vi "GDSProject_GetChidrenItemFromName.vi"(0 "ProjectItemToSearchFrom":refnum<vi>, 1 "ItemNameToSearchForInProjectTree":string, 2 "ItemToSearchForInProjectTreeBasedOnPath(used if wired)":path, 5 "error in (no error)":errorcluster) -> (14 "ProjectItemToSearchFromOut":refnum<vi>, 15 "ItemFound":bool, 16 "ProjectItemFound":refnum<vi>, 19 "error out":errorcluster)   [LabVIEW 2020]
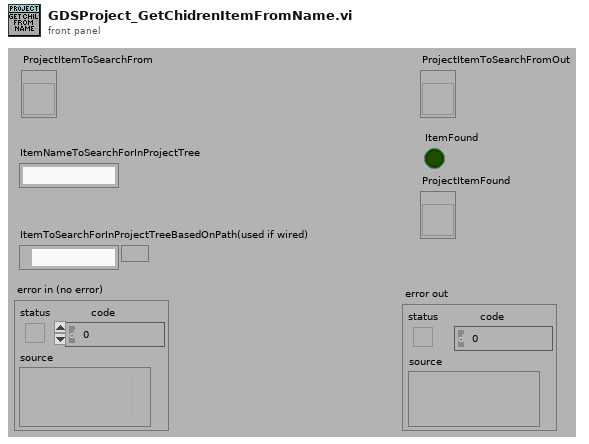
[diagram p1: front panel]
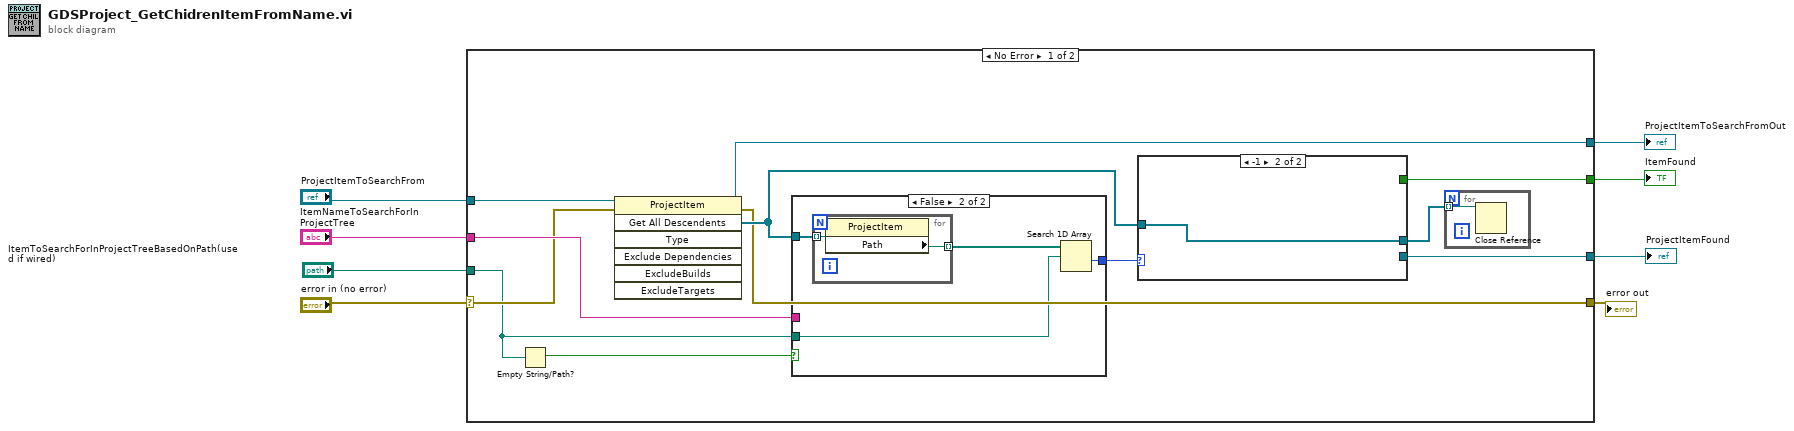
[diagram p0: block diagram]
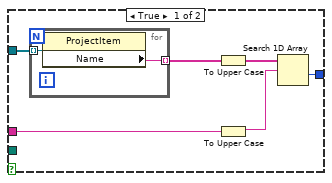
[diagram p2: hidden frame]
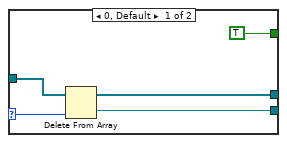
[diagram p3: hidden frame]
diagram:
  n1 = case shown="No Error" "error in (no error)" {
    selector: "error in (no error)" -> [w15 w43]
    tunnel: [w12 w43] -> w7
    tunnel: "ProjectItemToSearchFrom" -> [w20 w42]
    tunnel: "ItemNameToSearchForInProjectTree" -> [w19 _]
    tunnel: [w17 _] -> w4
    tunnel: [w16 w42] -> w3
    tunnel: [w13 _] -> w2
    tunnel: "ItemToSearchForInProjectTreeBasedOnPath(used if wired)" -> [w9 _]
    frame No Error {
      n2 = Empty String/Path?(string/path=w9) -> (empty?=w10:bool)
      n3 = invoke class="ProjectItem" method="Get All Descendents"(reference=w20, error in=w15) -> (reference out=w16:refnum<vi>, error out=w12:errorcluster, "All Descendents"=w14:refnum<vi>[])  [unwired: 5 in, 4 out]
      n4 = case shown="False" w10 {
        tunnel: w19 -> [w25 _]
        tunnel: [w22 w32] -> w18
        tunnel: w14 -> [w21 w31]
        tunnel: w9 -> [_ w29]
        frame True {
          n5 = for {
            tunnel: w21 -> [w28] mode=indexing
            tunnel: [w27] -> w26 mode=indexing
            n6 = property class="ProjectItem"(reference=w28) -> ("Name"=w27:string)  [unwired: 1 in, 2 out]
          }
          n7 = To Upper Case(1:w26) -> (0:w24:string[])
          n8 = To Upper Case(1:w25) -> (0:w23:string)
          n9 = Search 1D Array(1D array=w24, element=w23) -> (index of element=w22:i32)  [unwired: 1 in]
        }
        frame False {
          n10 = for {
            tunnel: w31 -> [w34] mode=indexing
            tunnel: [w33] -> w30 mode=indexing
            n11 = property class="ProjectItem"(reference=w34) -> ("Path"=w33:path)  [unwired: 1 in, 2 out]
          }
          n12 = Search 1D Array(1D array=w30, element=w29) -> (index of element=w32:i32)  [unwired: 1 in]
        }
      }
      n13 = case shown="-1" w18 {
        selector: w18 -> [w38 _]
        tunnel: [TRUE _] -> w17
        tunnel: w14 -> [w39 w41]
        tunnel: [w37 w41] -> w11
        tunnel: [w36 _] -> w13
        frame 0, Default {
          n14 = Delete From Array(array=w39, index=w38) -> (deleted portion=w36:refnum<vi>, array with subset deleted=w37:refnum<vi>[])  [unwired: 1 in]
        }
        frame -1 {
        }
      }
      n15 = for {
        tunnel: w11 -> [w35] mode=indexing
        n16 = Close Reference(reference=w35) -> ()  [unwired: 1 in, 1 out]
      }
    }
    frame Error {
    }
  }
  "error out" <- w7
  "ProjectItemToSearchFromOut" <- w3
  "ProjectItemFound" <- w2
  "ItemFound" <- w4
